vi "Merge.vi"(1 "背景":u8[][](array[numeric]), 2 "方块":u8[][](array[numeric]), 3 "point":cluster{"x":i16, "y":i16} caption="位置") -> (0 "输出":u8[][](array[numeric]))   [LabVIEW 2016]
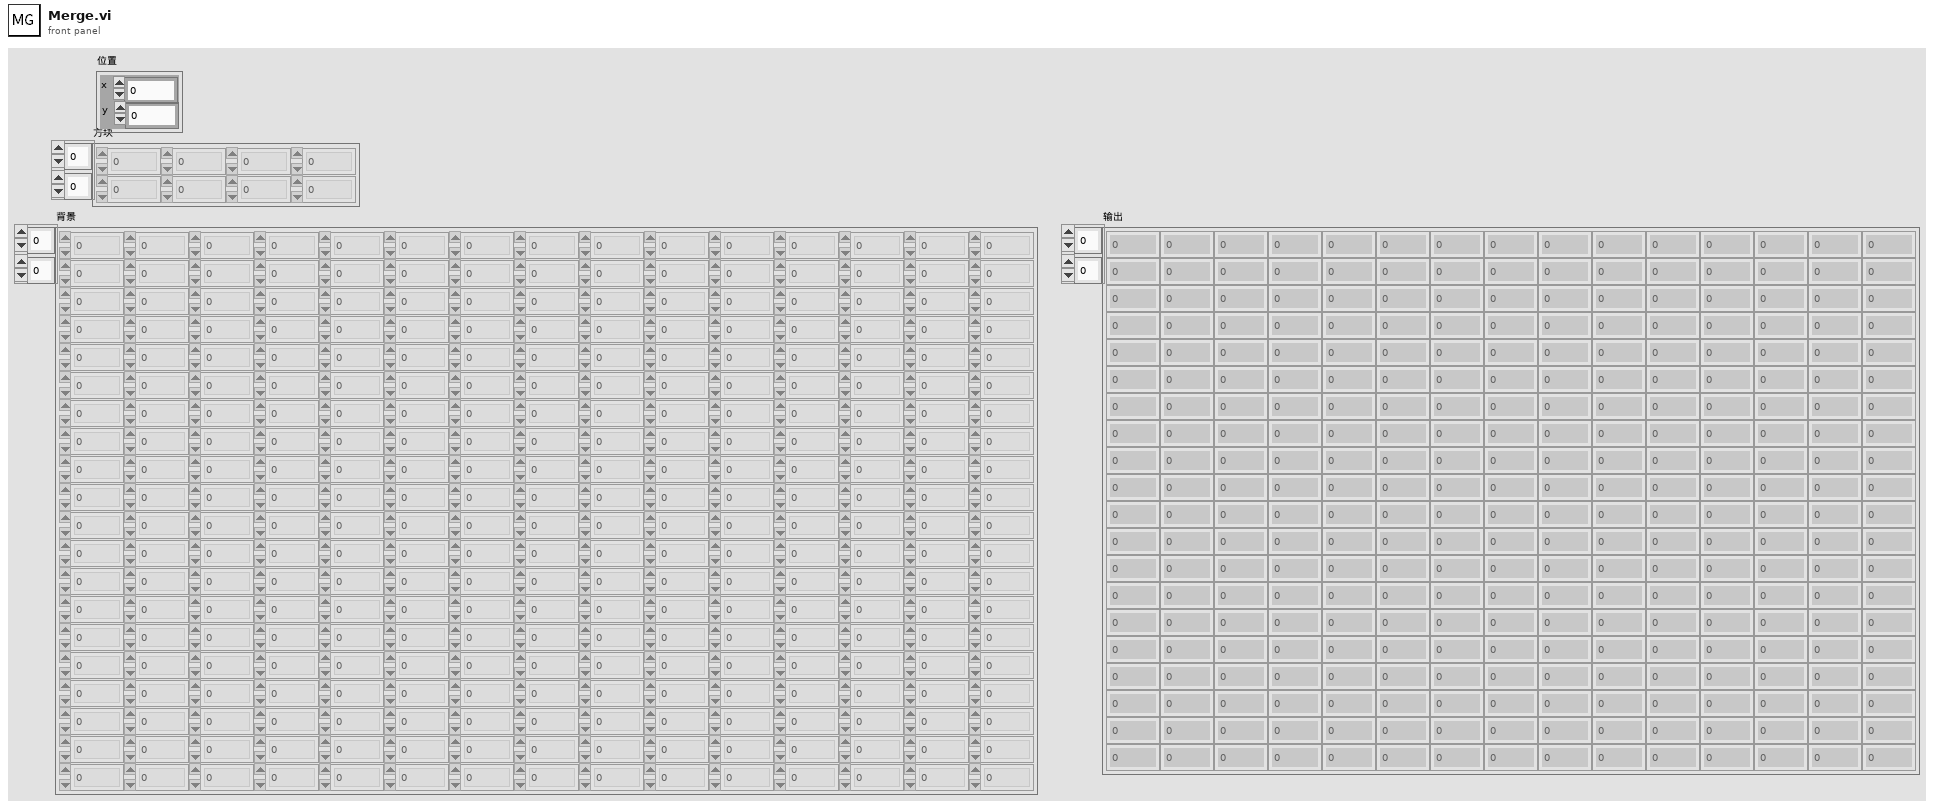
[diagram p1: front panel]
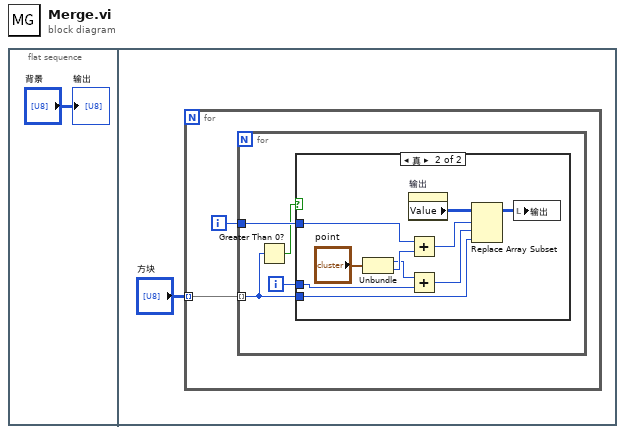
[diagram p0: block diagram]
diagram:
  n1 = flat-sequence {
    frame #0 {
      "输出" <- "背景"
    }
    frame #1 {
      n2 = for {
        tunnel: "方块" -> [w3] mode=indexing
        i -> [w4]
        n3 = for {
          tunnel: w4 -> [w8]
          tunnel: w3 -> [w6] mode=indexing
          i -> [w7]
          n4 = Greater Than 0?(x=w6) -> (x > 0?=w5:bool)
          n5 = case shown="真" w5 {
            tunnel: w8 -> [_ w17]
            tunnel: w7 -> [_ w13]
            tunnel: w6 -> [_ w11]
            frame False {
            }
            frame True {
              n6 = Unbundle("point") -> ("x"=w14:i16, "y"=w15:i16)
              n7 = property on="输出" class="Arr (严格)"() -> ("Value"=w10:u8[][])  [unwired: 2 in, 2 out]
              n8 = Add(x=w17, y=w15) -> (x+y=w16:i32)
              n9 = Add(x=w14, y=w13) -> (x+y=w12:i32)
              n10 = Replace Array Subset(array=w10, new element=w11, index (row)=w16, index (col)=w12) -> (w9:u8[][])
              n11 = local write "输出"(w9) -> ()
            }
          }
        }
      }
    }
  }
